vi "Omit App SSH Results.vi"(8 "error in (no error)":errorcluster, 9 "Message Data":variant, 10 "String":string) -> (0 "error out":errorcluster)   [LabVIEW 2024, in "User Interface.lvlib"]
uses:
  User Interface.lvlib
  Support/General Type Defs/Global Data.vi
  Support/General Type Defs/General Type Defs.lvlib
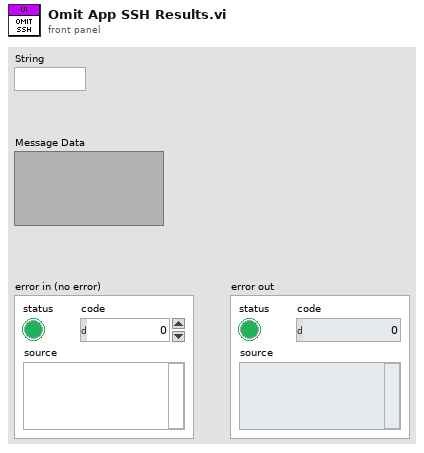
[diagram p1: front panel]
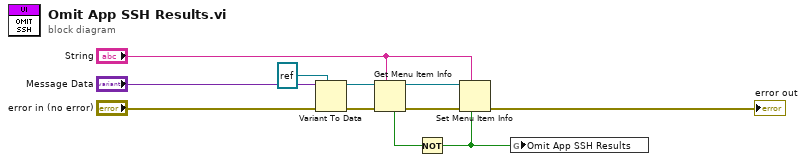
[diagram p0: block diagram]
diagram:
  n1 = Variant To Data(error in="error in (no error)", type=refnum<k9> refnum ("MenuRef"), Variant="Message Data") -> (data=w7:refnum<k9>, error out=w5:errorcluster)
  n2 = Get Menu Item Info(7:"String", 8:w5, 11:w7) -> (0:w3:errorcluster, 3:w4:refnum<k9>, 4:w2:bool)  [unwired: 4 out]
  n3 = Not(x=w2) -> (.not. x?=w1:bool)
  n4 = Set Menu Item Info(6:w1, 7:"String", 8:w3, 11:w4) -> (0:→"error out":errorcluster)  [unwired: 3 in, 1 out]
  n5 = global write "Global Data.vi" "Omit App SSH Results"(w1) -> ()
